vi "Handle.vi"(8 "Error In":errorcluster, 9 "Action":string, 10 "Values":dbl[](array[numeric]), 11 "object in":refnum<class "IHandler.lvclass">) -> (0 "Error Out":errorcluster, 2 "Return(DBL)":dbl, 3 "object out":refnum<class "IHandler.lvclass">)   [LabVIEW 2020, in "IHandler.lvclass"]
uses:
  IHandler.lvclass
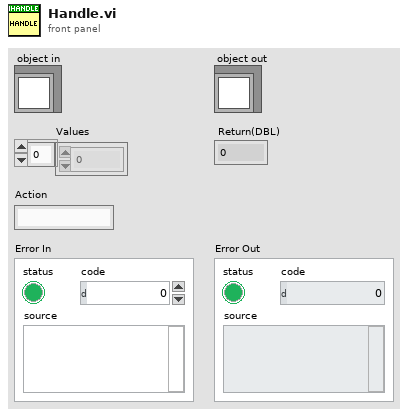
[diagram p1: front panel]
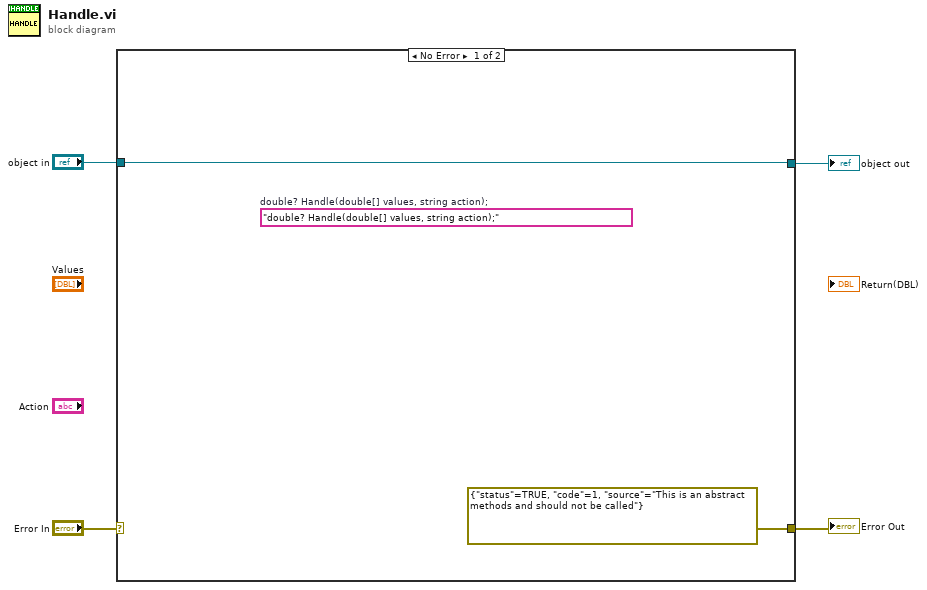
[diagram p0: block diagram]
diagram:
  n1 = case shown="No Error" "Error In" {
    selector: "Error In" -> [_ w8]
    tunnel: [errorcluster {"status"=TRUE, "code"=1, "source"="This is an abstract methods and should not be called"} ("error IO") w8] -> w3
    tunnel: [w6 w7] -> w1
    tunnel: "object in" -> [w6 w7]
    frame No Error {
      (unwired) "double? Handle(double[] values, string action);"  # double? Handle(double[] values, string action);
    }
    frame Error {
    }
  }
  "Error Out" <- w3
  "object out" <- w1
